vi "HammingWindow.vi"() -> ()   [LabVIEW 2009]
uses:
  <vilib>/imath/engines/lvmath2/RunTimeEngine/ErrorHandling/NIMS_Finalize Error.vi
  <vilib>/imath/engines/lvmath2/RunTimeEngine/Parser/MC_Version.vi
  <vilib>/imath/engines/lvmath2/RunTimeEngine/NodeEndStatement/NIMS_NodeEndStatement_Output.vi
  <instcachedir>/0/NIMS_NodeEndStatement_Output_53EC0D466D134D7ABD903AC30B43404B.lvgen/NIMS_NodeEndStatement_Output_53EC0D466D134D7ABD903AC30B43404B_001.vi
  <vilib>/imathl/engines/lvmath/Functions/Error Handling/Create Error.vi
  <vilib>/imath/engines/lvmath/Functions/Error Handling/MC_Error Cluster From Error Code.vi
  <vilib>/imath/engines/lvmath2/RunTimeEngine/BuiltInFunctions/win_hamming/NIMS_win_hamming.vi
  <vilib>/imath/engines/lvmath2/RunTimeEngine/BuiltInFunctions/freqzd/NIMS_freqzd().vi
  <vilib>/imath/engines/lvmath2/RunTimeEngine/BuiltInFunctions/win_hann2/NIMS_win_hann2.vi
panel:
  out "XY Graph":cluster{dbl[], dbl[]}[](graph)
  out "Waveform Graph 4":dbl[][](graph)
  in  "n1":dbl=256.0
  in  "N1":dbl=64.0
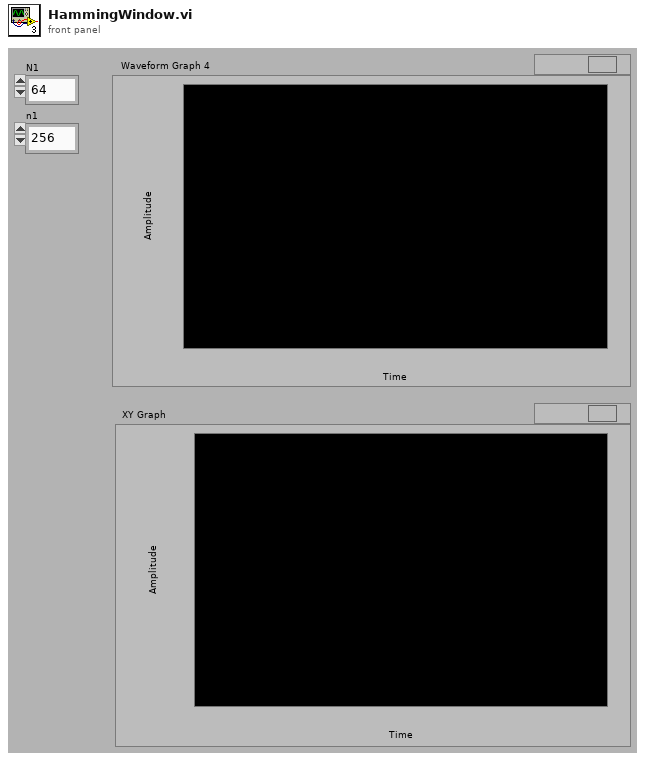
[diagram p1: front panel]
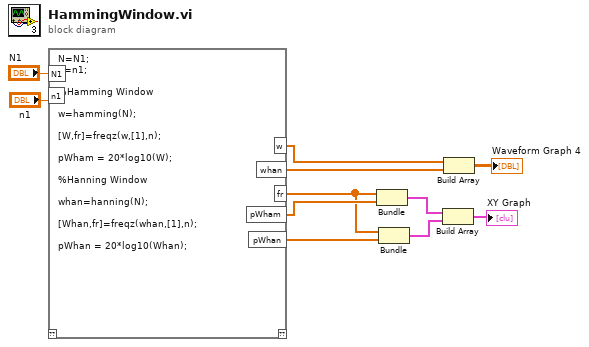
[diagram p0: block diagram]
diagram:
  n1 = mathscript code="N=N1;\nn=n1;\n\n%Hamming Window\n\nw=hamming(N);\n\n[W,fr]=freqz(w,[1],n);\n\npWham = 20*log10(W);\n\n%Hanning Window\n\nwhan=hanning(N);\n\n[Whan,fr]=freqz(whan,[1],n);\n\npWhan = 20*log10(Whan);"("N1"="N1", "n1"="n1") -> ("w"=w2:dbl[], "fr"=w7:dbl[], "pWham"=w9:dbl[], "whan"=w3:dbl[], "pWhan"=w8:dbl[])  [unwired: 1 in, 1 out]
  n2 = Bundle(w7, w9) -> (w6:cluster{dbl[], dbl[]})  [unwired: 1 in]
  n3 = Bundle(w7, w8) -> (w5:cluster{dbl[], dbl[]})  [unwired: 1 in]
  n4 = Build Array(w6, w5) -> (→"XY Graph":cluster{dbl[], dbl[]}[])
  n5 = Build Array(w2, w3) -> (→"Waveform Graph 4":dbl[][])
